vi "Check if Bounce is Necessary.vi"(8 "error in":errorcluster, 11 "Display State In":T1 caption="State") -> (0 "error out":errorcluster, 2 "Was Bounce Done?":bool, 3 "Display State Out 2":T1={"Numeric"=0.0, "Array of Button References"=[], "Space Between Menu Buttons"=3, "Number of Menu Buttons"=6, "Array of Button Names"=[], "Most Recent Vertical Position"=0, "This VI"=refnum, "Current Action"=enum."Not Moving", "Most Recent Distance Traveled"=0, "Method"=enum."Resize", "Data In"=0} caption="State")   [LabVIEW 2011, in "Sliding Menu Library.lvlib" / "Sliding Menu XControl.xctl"]
uses:
  Sliding Menu xControl/Sliding Menu XControl.xctl
  Sliding Menu xControl/Sliding Menu State.ctl
  Menu Button Library/Menu Button xControl/Menu Button xControl.xctl
  Sliding Menu Type Definitions/Current User Action.ctl
  Sliding Menu xControl/Sliding Menu Methods.ctl
  Sliding Menu xControl/Sliding Menu Data.ctl
  Sliding Menu Library.lvlib
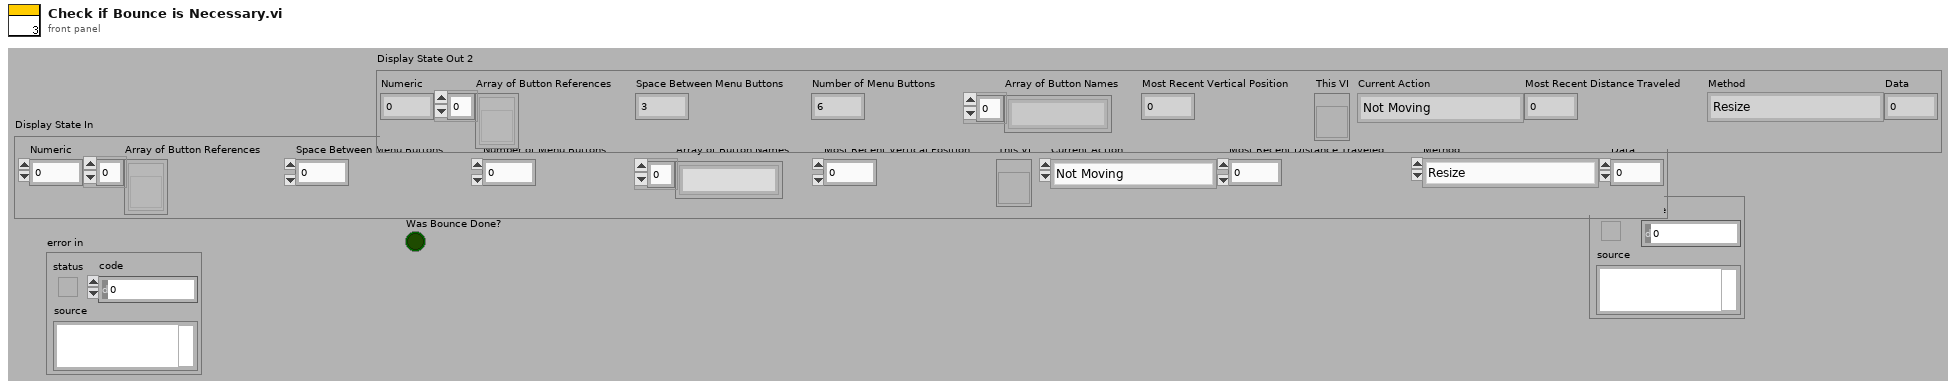
[diagram p1: front panel]
types:
  T1 = typedef "Sliding Menu Library.lvlib/Sliding Menu XControl.xctl/Sliding Menu State.ctl" = cluster{"Numeric":dbl, "Array of Button References":refnum<vi>[], "Space Between Menu Buttons":i32, "Number of Menu Buttons":i32, "Array of Button Names":string[], "Most Recent Vertical Position":i32, "This VI":refnum<vi>, "Current Action":T2, "Most Recent Distance Traveled":i32, "Method":T3, "Data In":T4}
  T2 = typedef "Sliding Menu Library.lvlib/Current User Action.ctl" = enum16{"Not Moving", "Mouse Down", "Mouse Up No Dragging", "Bounce Up Needed", "Bounce Down Needed", "Dragging", "Easing"}
  T3 = typedef "Sliding Menu Methods.ctl" = enum16{"Resize", "Move Up", "Move Down", "Move to 0"}
  T4 = typedef "Sliding Menu Library.lvlib/Sliding Menu XControl.xctl/Sliding Menu Data.ctl" = i32
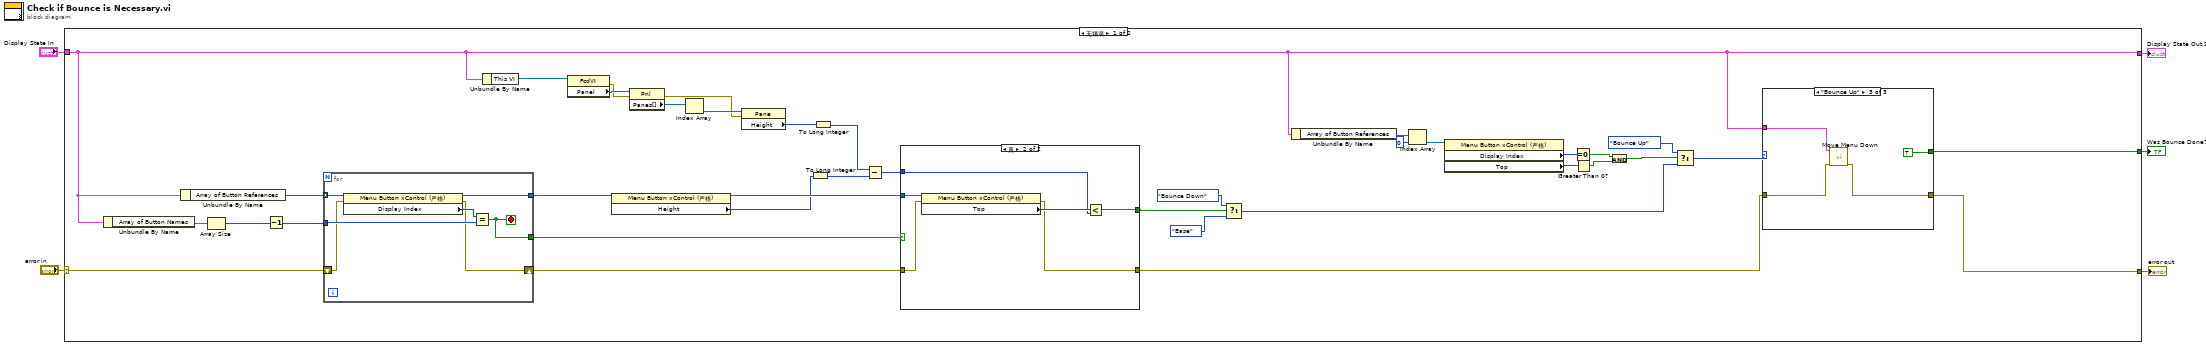
[diagram p0: block diagram]
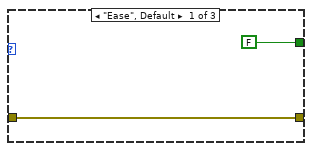
[diagram p2: hidden frame]
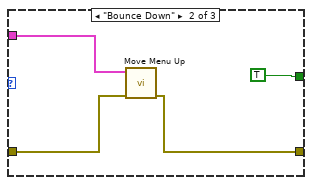
[diagram p3: hidden frame]
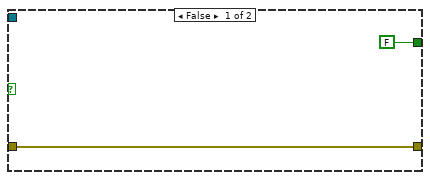
[diagram p4: hidden frame]
diagram:
  n1 = case shown="无错误" "error in" {
    selector: "error in" -> [w18 w69]
    tunnel: "Display State In" -> [w16 _]
    tunnel: [w15 w69] -> w5
    tunnel: [w16 _] -> w2
    tunnel: [w14 _] -> w1
    frame No Error {
      n2 = Unbundle By Name(w16) -> ("Array of Button Names"=w43:string[])
      n3 = Unbundle By Name(w16) -> ("Array of Button References"=w42:refnum<vi>[])
      n4 = Array Size(array=w43) -> (size(s)=w41:i32)
      n5 = Decrement(x=w41) -> (x-1=w40:i32)
      n6 = for {
        tunnel: w42 -> [w68] mode=indexing
        tunnel: w40 -> [w66]
        tunnel: [w65] -> w13
        shift-right: [w64] -> w7
        shift-left: w18 -> [w63]
        tunnel: [w62] -> w39
        stop <- w62 stop-if-true
        n7 = property class="Menu Button xControl (严格)"(reference=w68, error in=w63) -> (reference out=w65:refnum<vi>, error out=w64:errorcluster, "Display Index"=w67:i32)
        n8 = Equal?(x=w67, y=w66) -> (x = y?=w62:bool)
      }
      n9 = Unbundle By Name(w16) -> ("This VI"=w35:refnum<vi>)
      n10 = property class="FcdVI"(reference=w35) -> (error out=w20:errorcluster, "Panel"=w34:refnum<vi>)  [unwired: 1 in, 1 out]
      n11 = property class="Menu Button xControl (严格)"(reference=w13) -> (reference out=w12:refnum<vi>, "Height"=w8:u32)  [unwired: 1 in, 1 out]
      n12 = property class="Pnl"(reference=w34, error in=w20) -> (error out=w19:errorcluster, "Panes[]"=w33:refnum<vi>[])  [unwired: 1 out]
      n13 = Index Array(array=w33) -> (element=w32:refnum<vi>)  [unwired: 1 in]
      n14 = property class="Pane"(reference=w32, error in=w19) -> ("Height"=w31:u32)  [unwired: 2 out]
      n15 = To Long Integer(number=w8) -> (32bit integer=w9:i32)
      n16 = To Long Integer(number=w31) -> (32bit integer=w11:i32)
      n17 = Subtract(x=w11, y=w9) -> (x-y=w10:i32)
      n18 = case shown="真" w39 {
        tunnel: w12 -> [_ w61]
        tunnel: w7 -> [w55 w59]
        tunnel: [w55 w58] -> w6
        tunnel: [FALSE w57] -> w36
        tunnel: w10 -> [_ w56]
        frame False {
        }
        frame True {
          n19 = property class="Menu Button xControl (严格)"(reference=w61, error in=w59) -> (error out=w58:errorcluster, "Top"=w60:i32)  [unwired: 1 out]
          n20 = Less?(x=w60, y=w56) -> (x < y?=w57:bool)
        }
      }
      n21 = Select(t=enum16{"Ease", "Bounce Down", "Bounce Up"}."Bounce Down" ("Enum"), s=w36, f=enum16{"Ease", "Bounce Down", "Bounce Up"}."Ease" ("Enum")) -> (s? t:f=w22:enum16{"Ease", "Bounce Down", "Bounce Up"})
      n22 = Unbundle By Name(w16) -> ("Array of Button References"=w30:refnum<vi>[])
      n23 = Index Array(array=w30, index=0) -> (element=w29:refnum<vi>)
      n24 = property class="Menu Button xControl (严格)"(reference=w29) -> ("Display Index"=w28:i32, "Top"=w27:i32)  [unwired: 1 in, 2 out]
      n25 = Equal To 0?(x=w28) -> (x = 0?=w25:bool)
      n26 = Greater Than 0?(x=w27) -> (x > 0?=w24:bool)
      n27 = And(x=w25, y=w24) -> (x .and. y?=w23:bool)
      n28 = Select(t=enum16{"Ease", "Bounce Down", "Bounce Up"}."Bounce Up" ("Enum"), s=w23, f=w22) -> (s? t:f=w17:enum16{"Ease", "Bounce Down", "Bounce Up"})
      n29 = case shown="\"Bounce Up\"" w17 {
        tunnel: w6 -> [w45 w48 w52]
        tunnel: w16 -> [_ w49 w53]
        tunnel: [w45 w46 w51] -> w15
        tunnel: [FALSE TRUE TRUE] -> w14
        frame "Ease", Default {
        }
        frame "Bounce Down" {
          n30 = call "Move Menu Up.vi"("error in (no error)"=w48, "Display State In"=w49) -> ("error out"=w46:errorcluster)  [unwired: 8 in, 1 out]
        }
        frame "Bounce Up" {
          n31 = call "Move Menu Down.vi"("error in (no error)"=w52, "Display State In"=w53) -> ("error out"=w51:errorcluster)  [unwired: 8 in, 1 out]
        }
      }
    }
    frame Error {
    }
  }
  "error out" <- w5
  "Display State Out 2" <- w2
  "Was Bounce Done?" <- w1
